vi "Find D Matrix.vi"(1 "Complex FT":cdb[][](array[numeric]) format="%.2f") -> (0 "Intensity Graph":dbl[][](graph))   [LabVIEW 2024]
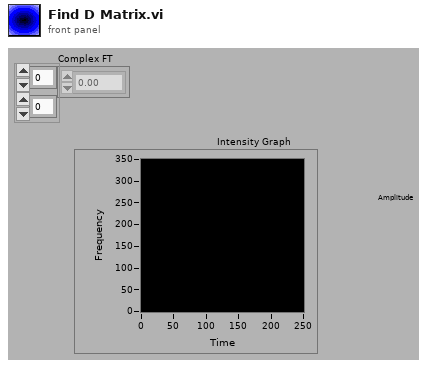
[diagram p1: front panel]
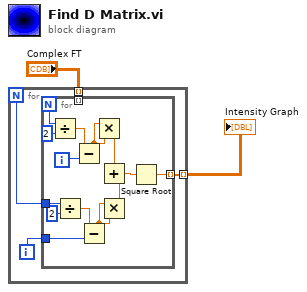
[diagram p0: block diagram]
diagram:
  n1 = for {
    N -> [w4]
    tunnel: "Complex FT" -> [w6] mode=indexing
    tunnel: [w3] -> w2 mode=indexing
    i -> [w5]
    n2 = for {
      N -> [w19]
      tunnel: w6 -> [_] mode=indexing
      tunnel: w5 -> [w12]
      tunnel: w4 -> [w11]
      tunnel: [w7] -> w3 mode=indexing
      i -> [w20]
      n3 = Divide(x=w19, y=2) -> (x/y=w17:dbl)
      n4 = Divide(x=w11, y=2) -> (x/y=w14:dbl)
      n5 = Subtract(x=w17, y=w20) -> (x-y=w16:dbl)
      n6 = Subtract(x=w14, y=w12) -> (x-y=w15:dbl)
      n7 = Multiply(x=w16, y=w16) -> (x*y=w10:dbl)
      n8 = Multiply(x=w15, y=w15) -> (x*y=w9:dbl)
      n9 = Add(x=w10, y=w9) -> (x+y=w8:dbl)
      n10 = Square Root(x=w8) -> (sqrt(x)=w7:dbl)
    }
  }
  "Intensity Graph" <- w2
